vi "Read Item Indent.vi"(11 "BetterTreeItem in":refnum<class "BetterItem.lvclass">) -> (2 "Item Indent":i32, 3 "BetterTreeItem out":refnum<class "BetterItem.lvclass">)   [LabVIEW 2020, in "BetterDragAndDrop.lvlib" / "BetterItem.lvclass"]
uses:
  BetterItem.lvclass
  BetterItem.lvclass/BetterItem.ctl
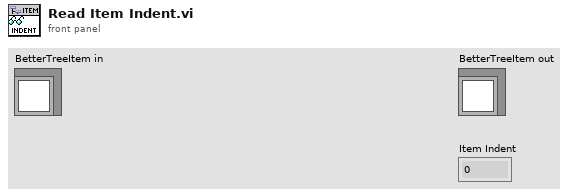
[diagram p1: front panel]
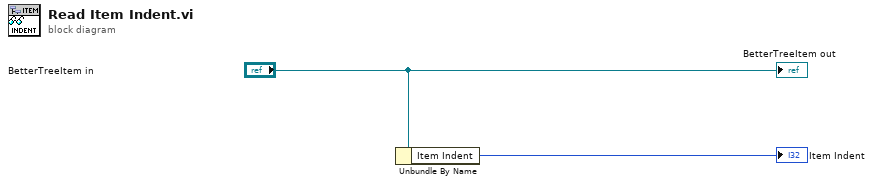
[diagram p0: block diagram]
diagram:
  n1 = Unbundle By Name("BetterTreeItem in") -> ("Item Indent"=→"Item Indent":i32)
  "BetterTreeItem out" <- "BetterTreeItem in"
